vi "Change Use Default Limits.vi"(8 "error in (no error)":errorcluster, 10 "Use Default Limits":bool, 11 "Numeric Data Type in":refnum<class "Numeric Data Type.lvclass">) -> (0 "error out":errorcluster, 3 "Numeric Data Type out":refnum<class "Numeric Data Type.lvclass">)   [LabVIEW 2018, in "Numeric Data Type.lvclass"]
uses:
  Numeric Data Type.lvclass
  Numeric Data Type.lvclass/Numeric Data Type.ctl
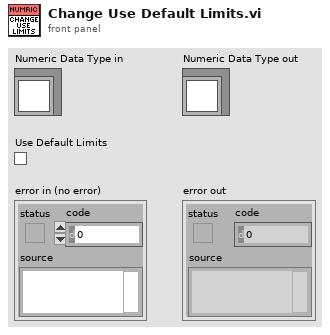
[diagram p1: front panel]
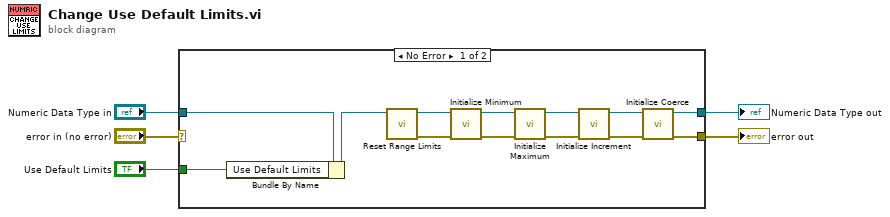
[diagram p0: block diagram]
diagram:
  n1 = case shown="No Error" "error in (no error)" {
    selector: "error in (no error)" -> [_ w20]
    tunnel: [w10 w20] -> w4
    tunnel: [w12 w19] -> w2
    tunnel: "Numeric Data Type in" -> [w18 w19]
    tunnel: "Use Default Limits" -> [w9 _]
    frame No Error {
      n2 = Bundle By Name(cluster=w18, "Use Default Limits"=w9) -> (w8:refnum<class "Numeric Data Type.lvclass">)
      n3 = call "Reset Range Limits.vi"("Numeric Data Type in"=w8) -> ("error out"=w6:errorcluster, "Numeric Data Type out"=w7:refnum<class "Numeric Data Type.lvclass">)  [unwired: 9 in]
      n4 = call "Initialize Minimum.vi"("error in (no error)"=w6, "Numeric Data Type in"=w7) -> ("error out"=w16:errorcluster, "Numeric Data Type (dup)"=w17:refnum<class "Numeric Data Type.lvclass">)  [unwired: 8 in]
      n5 = call "Initialize Maximum.vi"("error in (no error)"=w16, "Numeric Data Type in"=w17) -> ("error out"=w14:errorcluster, "Numeric Data Type (dup)"=w15:refnum<class "Numeric Data Type.lvclass">)  [unwired: 8 in]
      n6 = call "Initialize Increment.vi"("error in (no error)"=w14, "Numeric Data Type in"=w15) -> ("error out"=w11:errorcluster, "Numeric Data Type (dup)"=w13:refnum<class "Numeric Data Type.lvclass">)  [unwired: 8 in]
      n7 = call "Initialize Coerce.vi"("error in (no error)"=w11, "Numeric Data Type in"=w13) -> ("error out"=w10:errorcluster, "Numeric Data Type (dup)"=w12:refnum<class "Numeric Data Type.lvclass">)  [unwired: 8 in]
    }
    frame Error {
    }
  }
  "error out" <- w4
  "Numeric Data Type out" <- w2
